vi "Write STL file (binary format).vi"(2 "STL header (must be 80 bytes)":string="STL binary output from Paul Nathan's LabVIEW code.                              ", 3 "Panel triangles array":T1[](array[typedef]), 4 "STL file path":path) -> (0 "Error out":errorcluster)   [LabVIEW 2017]
doc: "Note: The STL file must be in binary format, not ASCII."
uses:
  ctls/Triangle panel.ctl
panel:
  # "PN 21/11/17"
  # "Vertices"
  # "Edges"
  # "Unit normal"
  # "Control point"
  # "Edge\nlinks \n(tri index)"
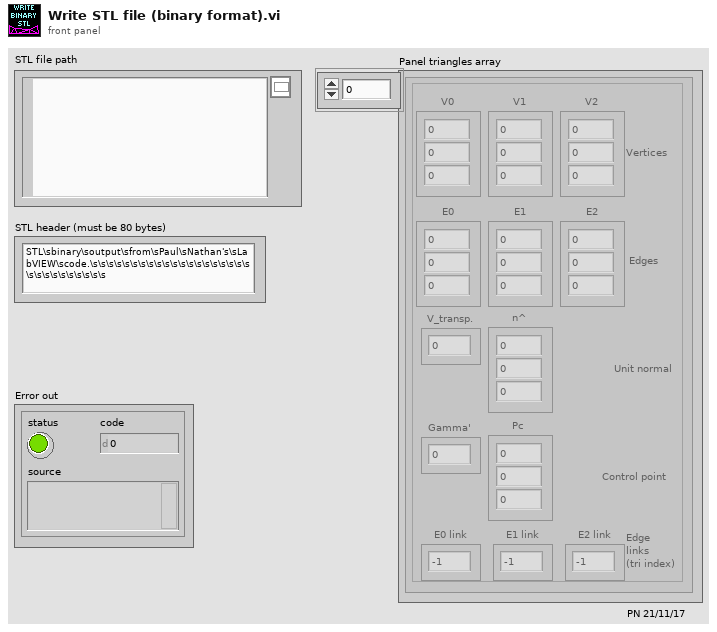
[diagram p1: front panel]
types:
  T1 = typedef "Triangle panel.ctl" = cluster{"V0":sgl[], "V1":sgl[], "V2":sgl[], "E0":sgl[], "E1":sgl[], "E2":sgl[], "n^":sgl[], "Pc":sgl[], "Gamma'":sgl, "V_transp.":sgl, "E0 link":i32, "E1 link":i32, "E2 link":i32}
  T2 = enum16{"big-endian, network order", "native, host order", "little-endian"}
  T3 = enum16{"open", "replace", "create", "open or create", "replace or create", "replace or create with confirmation"}
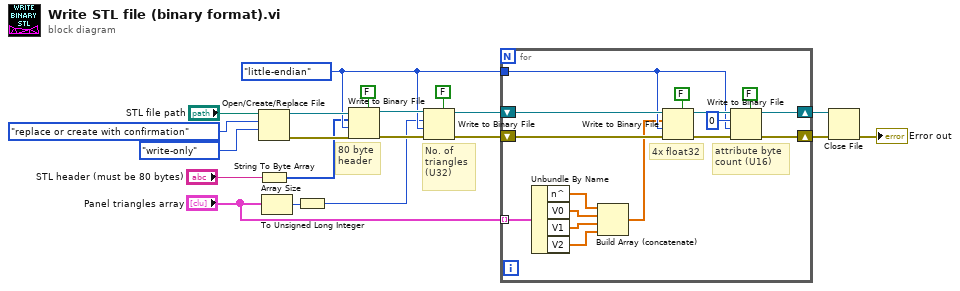
[diagram p0: block diagram]
diagram:
  w9 = T2."little-endian" ("byte order (0:big-endian, network order)")
  # "No. of triangles (U32)"
  # "80 byte header"
  n1 = Open/Create/Replace File(file path (use dialog)="STL file path", operation (0:open)=T3."replace or create with confirmation", access (0:read/write)=enum16{"read/write", "read-only", "write-only"}."write-only") -> (refnum out=w18:refnum<file>, error out=w17:errorcluster)  [unwired: 3 in, 1 out]
  n2 = String To Byte Array(string="STL header (must be 80 bytes)") -> (unsigned byte array=w5:u8[])
  n3 = Array Size(array="Panel triangles array") -> (size(s)=w3:i32)
  n4 = To Unsigned Long Integer(number=w3) -> (unsigned 32bit integer=w2:u32)
  n5 = Write to Binary File(file (use dialog)=w18, data=w5, error in=w17, 5:FALSE ("prepend array or string size? (T)"), 9:w9) -> (refnum out=w16:refnum<file>, error out=w15:errorcluster)  [unwired: 1 in, 1 out]
  n6 = Write to Binary File(file (use dialog)=w16, data=w2, error in=w15, 5:FALSE ("prepend array or string size? (T)"), 9:w9) -> (refnum out=w13:refnum<file>, error out=w14:errorcluster)  [unwired: 1 in, 1 out]
  n7 = for {
    shift-right: [w30] -> w11
    shift-left: w14 -> [w35]
    shift-right: [w31] -> w12
    shift-left: w13 -> [w36]
    tunnel: w9 -> [w29]
    tunnel: "Panel triangles array" -> [w28] mode=indexing
    # "4x float32"
    # "attribute byte count (U16)"
    n8 = Unbundle By Name(w28) -> ("n^"=w25:sgl[], "V0"=w24:sgl[], "V1"=w23:sgl[], "V2"=w22:sgl[])
    n9 = Build Array (concatenate)(w25, w24, w23, w22) -> (w21:sgl[])
    n10 = Write to Binary File(file (use dialog)=w36, data=w21, error in=w35, 5:FALSE ("prepend array or string size? (T)"), 9:w29) -> (refnum out=w32:refnum<file>, error out=w33:errorcluster)  [unwired: 1 in, 1 out]
    n11 = Write to Binary File(file (use dialog)=w32, data=u16 0 ("count (1)"), error in=w33, 5:FALSE ("prepend array or string size? (T)"), 9:w29) -> (refnum out=w31:refnum<file>, error out=w30:errorcluster)  [unwired: 1 in, 1 out]
  }
  n12 = Close File(refnum=w12, error in=w11) -> (error out=→"Error out":errorcluster)  [unwired: 1 out]
